vi "DSF.Engine.Execution.Transfer.Validate Configuration.vi"(8 "error in (no error)":errorcluster, 11 "Transfer in":refnum<class "DSF.Engine.Execution.Transfer.lvclass">) -> (0 "error out":errorcluster, 3 "Transfer out":refnum<class "DSF.Engine.Execution.Transfer.lvclass">)   [LabVIEW 2016, in "DSF.Engine.lvlib" / "DSF.Engine.Execution.Transfer.lvclass"]
uses:
  DSF.Engine.Execution.Transfer.lvclass
  Shared/Typedefs/DSF.Shared.Typedefs.Configuration.Transfer.Channel Parameters.ctl
  Shared/Typedefs/DSF.Shared.Typedefs.Data Type.ctl
  DSF.Shared.lvlib
panel:
  out "invalid index":i32
  out "valid?":bool
  out "Channels Configuration out":T1[](array[typedef]) {"offset" format="%d bytes"}
  in  "Channels Configuration in":T1[](array[typedef]) {"offset" format="%d bytes"}
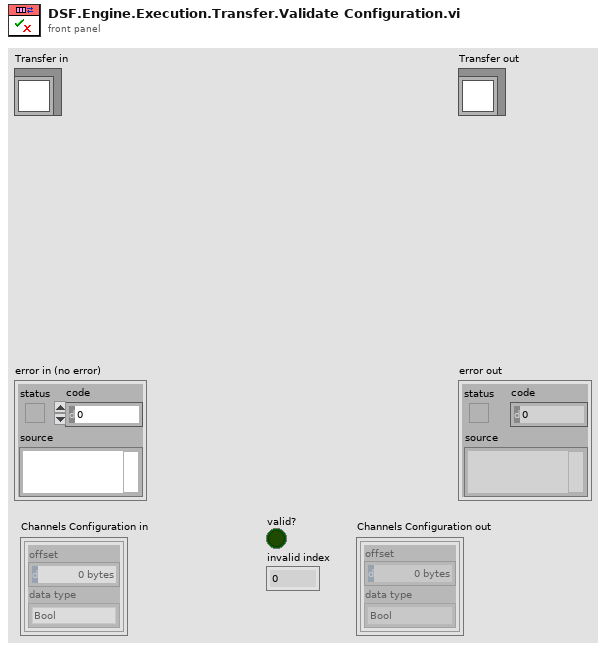
[diagram p1: front panel]
types:
  T1 = typedef "DSF.Shared.lvlib/DSF.Shared.Typedefs.Configuration.Transfer.Channel Parameters.ctl" = cluster{"offset":u64, "data type":T2}
  T2 = typedef "DSF.Shared.lvlib/DSF.Shared.Typedefs.Data Type.ctl" = enum8{"Bool", "SGL", "DBL", "I8", "I16", "I32", "I64", "U8", "U16", "U32", "U64"}
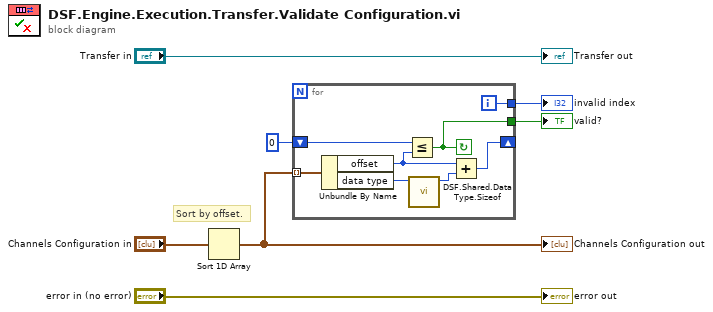
[diagram p0: block diagram]
diagram:
  # "Sort by offset."
  n1 = Sort 1D Array(array="Channels Configuration in") -> (sorted array=w5:T1[])
  "Channels Configuration out" <- w5
  n2 = for {
    tunnel: w5 -> [w15] mode=indexing
    shift-right: [w10] -> _
    shift-left: u64 0 ("offset") -> [w14]
    tunnel: [w9] -> w3
    tunnel: [w8] -> w4
    i -> [w9]
    stop <- w8 continue-if-true
    n3 = Unbundle By Name(w15) -> ("offset"=w12:u64, "data type"=w13:T2)
    n4 = Less Or Equal?(x=w14, y=w12) -> (x <= y?=w8:bool)
    n5 = call "DSF.Shared.Data Type.Sizeof.vi"("data type"=w13) -> ("size in bytes"=w11:u64)  [unwired: 9 in, 1 out]
    n6 = Add(x=w12, y=w11) -> (x+y=w10:u64)
  }
  "valid?" <- w4
  "invalid index" <- w3
  "error out" <- "error in (no error)"
  "Transfer out" <- "Transfer in"
